vi "SUB-BLE Rx data (Debug)-CDC_KH.vi"(8 "data in":u8[](array[numeric]) format="%2x") -> (2 "CDC debug":T1 caption="CDC Debugging data" {"Right Wing-C, C6/C0" format="%#.9f"; "Right Wing-B, C5/C0" format="%#.9f"; "Right Wing-A, C4/C0" format="%#.9f"; "Left Wing-C, C3/C0" format="%#.9f"; "Left Wing-B, C2/C0" format="%#.9f"; "Left Wing-A, C1/C0" format="%#.9f"}, 3 "CDC mon":T1 caption="CDC Monitoring data" {"Right Wing-C, C6/C0" format="%#.9f"; "Right Wing-B, C5/C0" format="%#.9f"; "Right Wing-A, C4/C0" format="%#.9f"; "Left Wing-C, C3/C0" format="%#.9f"; "Left Wing-B, C2/C0" format="%#.9f"; "Left Wing-A, C1/C0" format="%#.9f"})   [LabVIEW 2015]
doc: "Use this template to create an application that executes repeatedly until you click the Stop button. This template polls the state of the Stop button and does not use events. Use the Top-Level Application template (not available in the Base package) to create a single-loop application with event handling."
panel:
  out "BLE Packet (buf)":u8[](array[numeric])
  out "BLE Packet (data)":u8[](array[numeric])
  # "BLE 수신 데이터를 처리: Debugging data"
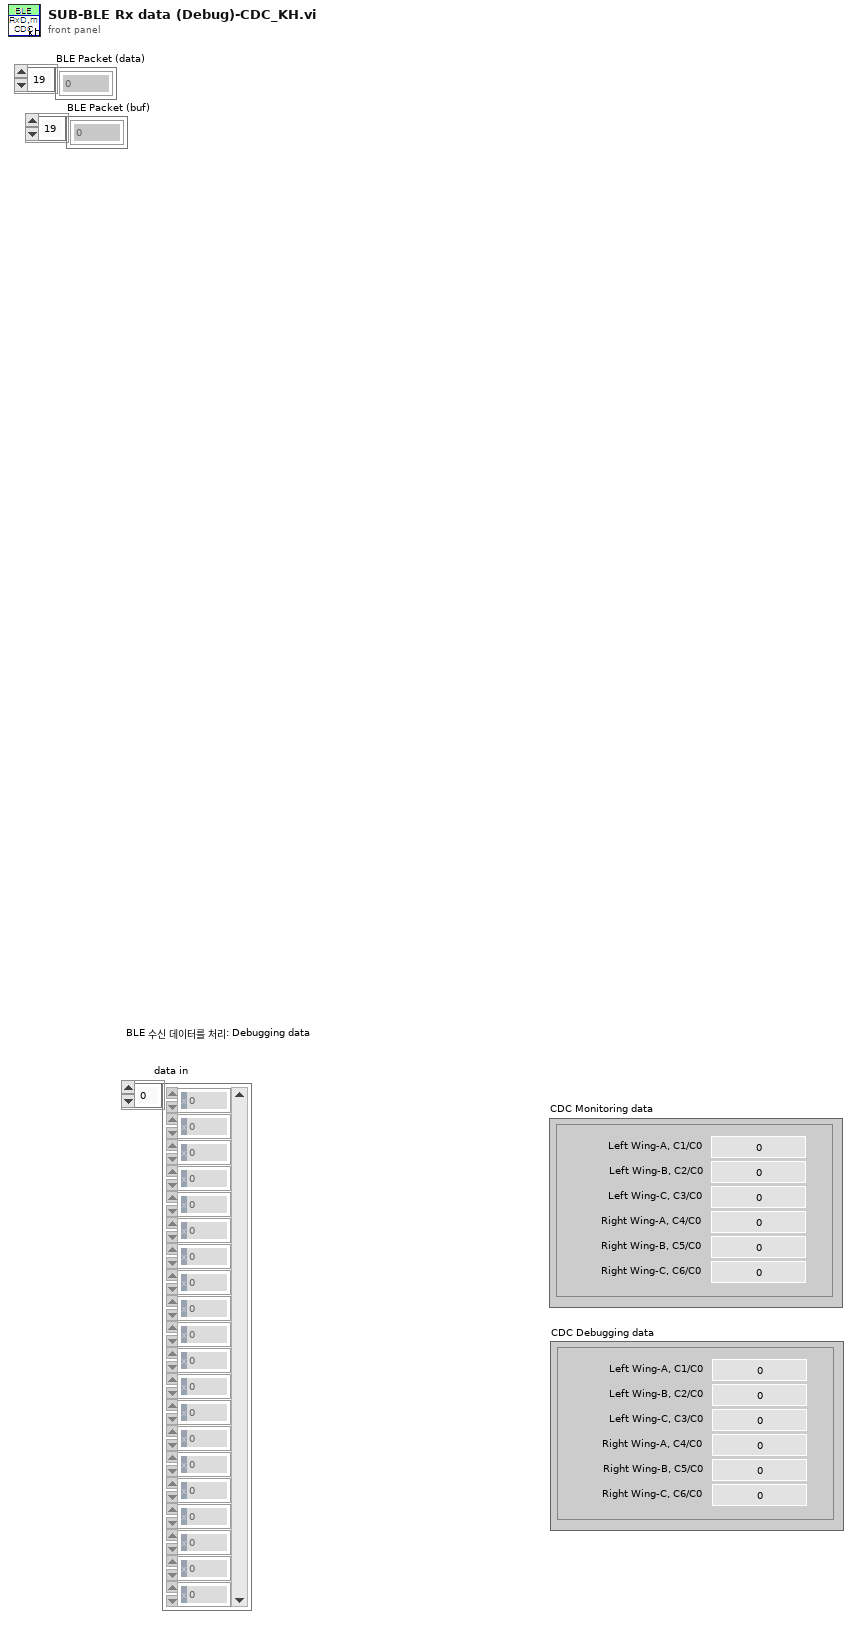
[diagram p1: front panel]
types:
  T1 = typedef "컨트롤-CDC data.ctl" = cluster{"Left Wing-A, C1/C0":dbl, "Left Wing-B, C2/C0":dbl, "Left Wing-C, C3/C0":dbl, "Right Wing-A, C4/C0":dbl, "Right Wing-B, C5/C0":dbl, "Right Wing-C, C6/C0":dbl}
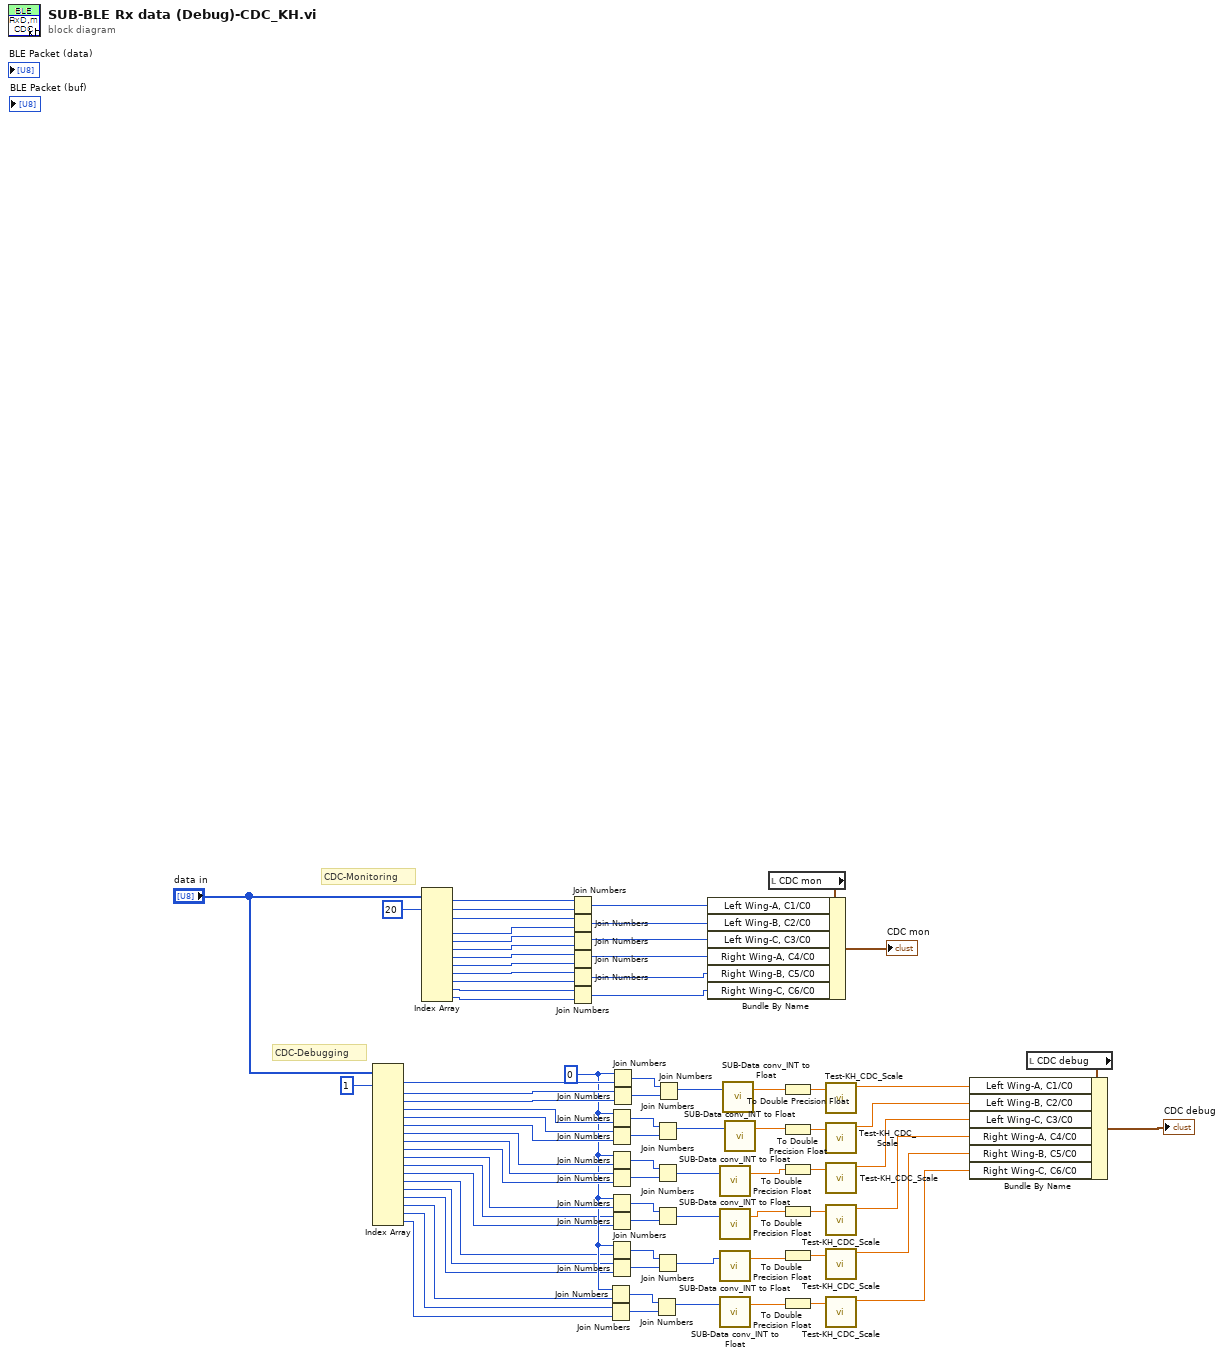
[diagram p0: block diagram]
diagram:
  w33 = u8 0 ("hi")
  # "CDC-Debugging"
  # "CDC-Monitoring"
  n1 = Index Array(array="data in", index #1=1 ("인덱스")) -> (element #1=w55:u8, element #2=w54:u8, element #3=w53:u8, element #4=w40:u8, element #5=w39:u8, element #6=w38:u8, element #7=w37:u8, element #8=w36:u8, element #9=w35:u8, element #10=w34:u8, element #11=w32:u8, element #12=w31:u8, element #13=w30:u8, element #14=w29:u8, element #15=w28:u8, element #16=w27:u8, element #17=w26:u8, element #18=w25:u8)  [unwired: 17 in]
  n2 = Index Array(array="data in", index #1=20 ("인덱스")) -> (element #1=w78:u8, element #2=w77:u8, element #3=w76:u8, element #4=w75:u8, element #5=w74:u8, element #6=w73:u8, element #7=w72:u8, element #8=w71:u8, element #9=w70:u8, element #10=w69:u8, element #11=w68:u8, element #12=w67:u8)  [unwired: 11 in]
  n3 = Join Numbers(hi=w78, lo=w77) -> ((hi.lo)=w65:u16)
  n4 = Join Numbers(hi=w76, lo=w75) -> ((hi.lo)=w64:u16)
  n5 = Join Numbers(hi=w74, lo=w73) -> ((hi.lo)=w63:u16)
  n6 = Join Numbers(hi=w72, lo=w71) -> ((hi.lo)=w62:u16)
  n7 = Join Numbers(hi=w70, lo=w69) -> ((hi.lo)=w61:u16)
  n8 = Join Numbers(hi=w68, lo=w67) -> ((hi.lo)=w60:u16)
  n9 = Join Numbers(hi=w33, lo=w27) -> ((hi.lo)=w42:u16)
  n10 = Join Numbers(hi=w26, lo=w25) -> ((hi.lo)=w41:u16)
  n11 = Join Numbers(hi=w33, lo=w40) -> ((hi.lo)=w50:u16)
  n12 = Join Numbers(hi=w39, lo=w38) -> ((hi.lo)=w49:u16)
  n13 = Join Numbers(hi=w33, lo=w37) -> ((hi.lo)=w47:u16)
  n14 = Join Numbers(hi=w36, lo=w35) -> ((hi.lo)=w48:u16)
  n15 = Join Numbers(hi=w33, lo=w34) -> ((hi.lo)=w46:u16)
  n16 = Join Numbers(hi=w32, lo=w31) -> ((hi.lo)=w45:u16)
  n17 = Join Numbers(hi=w33, lo=w30) -> ((hi.lo)=w43:u16)
  n18 = Join Numbers(hi=w29, lo=w28) -> ((hi.lo)=w44:u16)
  n19 = Join Numbers(hi=w33, lo=w55) -> ((hi.lo)=w51:u16)
  n20 = Join Numbers(hi=w54, lo=w53) -> ((hi.lo)=w52:u16)
  n21 = Join Numbers(hi=w42, lo=w41) -> ((hi.lo)=w23:u32)
  n22 = Join Numbers(hi=w50, lo=w49) -> ((hi.lo)=w20:u32)
  n23 = Join Numbers(hi=w47, lo=w48) -> ((hi.lo)=w21:u32)
  n24 = Join Numbers(hi=w46, lo=w45) -> ((hi.lo)=w22:u32)
  n25 = Join Numbers(hi=w43, lo=w44) -> ((hi.lo)=w24:u32)
  n26 = Join Numbers(hi=w51, lo=w52) -> ((hi.lo)=w19:u32)
  n27 = call "SUB-Data conv_INT to Float.vi"("U32"=w21) -> ("FP32"=w9:sgl)  [unwired: 2 in]
  n28 = call "SUB-Data conv_INT to Float.vi"("U32"=w22) -> ("FP32"=w8:sgl)  [unwired: 2 in]
  n29 = call "SUB-Data conv_INT to Float.vi"("U32"=w24) -> ("FP32"=w7:sgl)  [unwired: 2 in]
  n30 = call "SUB-Data conv_INT to Float.vi"("U32"=w23) -> ("FP32"=w6:sgl)  [unwired: 2 in]
  n31 = call "SUB-Data conv_INT to Float.vi"("U32"=w19) -> ("FP32"=w18:sgl)  [unwired: 2 in]
  n32 = call "SUB-Data conv_INT to Float.vi"("U32"=w20) -> ("FP32"=w10:sgl)  [unwired: 2 in]
  n33 = local read "CDC mon"() -> (w80:T1)
  n34 = Bundle By Name(cluster=w80, "Left Wing-A, C1/C0"=w65, "Left Wing-B, C2/C0"=w64, "Left Wing-C, C3/C0"=w63, "Right Wing-A, C4/C0"=w62, "Right Wing-B, C5/C0"=w61, "Right Wing-C, C6/C0"=w60) -> (→"CDC mon":T1)
  n35 = To Double Precision Float(number=w18) -> (double precision float=w16:dbl)
  n36 = To Double Precision Float(number=w10) -> (double precision float=w15:dbl)
  n37 = To Double Precision Float(number=w9) -> (double precision float=w14:dbl)
  n38 = To Double Precision Float(number=w8) -> (double precision float=w13:dbl)
  n39 = To Double Precision Float(number=w7) -> (double precision float=w12:dbl)
  n40 = To Double Precision Float(number=w6) -> (double precision float=w11:dbl)
  n41 = call "Test-KH_CDC_Scale.vi"("r"=w16) -> ("2byte"=w17:dbl)  [unwired: 10 in]
  n42 = call "Test-KH_CDC_Scale.vi"("r"=w15) -> ("2byte"=w5:dbl)  [unwired: 10 in]
  n43 = call "Test-KH_CDC_Scale.vi"("r"=w14) -> ("2byte"=w4:dbl)  [unwired: 10 in]
  n44 = call "Test-KH_CDC_Scale.vi"("r"=w13) -> ("2byte"=w3:dbl)  [unwired: 10 in]
  n45 = call "Test-KH_CDC_Scale.vi"("r"=w12) -> ("2byte"=w2:dbl)  [unwired: 10 in]
  n46 = call "Test-KH_CDC_Scale.vi"("r"=w11) -> ("2byte"=w1:dbl)  [unwired: 10 in]
  n47 = local read "CDC debug"() -> (w58:T1)
  n48 = Bundle By Name(cluster=w58, "Left Wing-A, C1/C0"=w17, "Left Wing-B, C2/C0"=w5, "Left Wing-C, C3/C0"=w4, "Right Wing-A, C4/C0"=w3, "Right Wing-B, C5/C0"=w2, "Right Wing-C, C6/C0"=w1) -> (→"CDC debug":T1)
